vi "Hysteresis-Polynom2Preisach.vi"(9 "Polynomial Coefficients bwd":dbl[](array[numeric]), 10 "relative Range":dbl, 11 "Polynomial Coefficients fwd":dbl[](array[numeric])) -> (3 "Preisach":dbl[](array[numeric]))   [LabVIEW 2016]
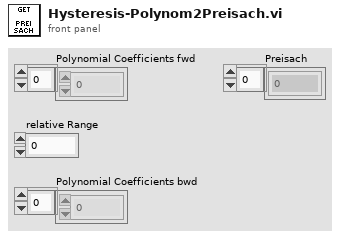
[diagram p1: front panel]
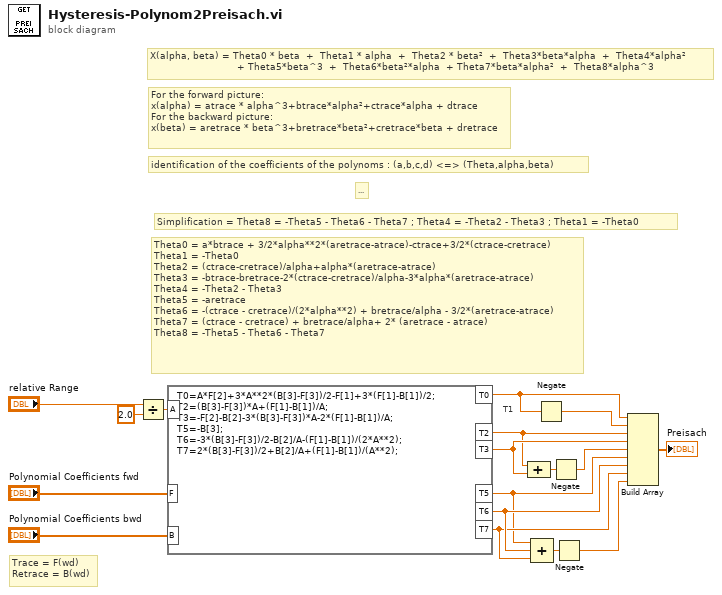
[diagram p0: block diagram]
diagram:
  # "Simplification = Theta8 = -Theta5 - Theta6 - Theta7 ; Theta4 = -Theta2 - Theta3 ; Theta1 = -Theta0"
  # "..."
  # "X(alpha, beta) = Theta0 * beta  +  Theta1 * alpha  +  Theta2 * beta²  +  Theta3*beta*alpha  +  Theta4*alpha² \n                             + Theta5*beta^3  +  Theta6*beta²*alpha  + Theta7*beta*alpha²  +  Theta8*alpha^3"
  # "identification of the coefficients of the polynoms : (a,b,c,d) <=> (Theta,alpha,beta)"
  # "For the forward picture:\nx(alpha) = atrace * alpha^3+btrace*alpha²+ctrace*alpha + dtrace\nFor the backward picture:\nx(beta) = aretrace * beta^3+bretrace*beta²+cretrace*beta + dretrace"
  # "Trace = F(wd)\nRetrace = B(wd)"
  # "T1"
  # "Theta0 = a*btrace + 3/2*alpha**2*(aretrace-atrace)-ctrace+3/2*(ctrace-cretrace)\nTheta1 = -Theta0\nTheta2 = (ctrace-cretrace)/alpha+alpha*(aretrace-atrace)\nTheta3 = -btrace-bretrace-2*(ctrace-cretrace)/alpha-3*alpha*(aretrace-atrace)\nTheta4 = -Theta2 - Theta3\nTheta5 = -aretrace\nTheta6 = -(ctrace - cretrace)/(2*alpha**2) + bretrace/alpha - 3/2*(aretrace-atrace)\nTheta7 = (ctrace - cretrace) + bretrace/alpha+ 2* (aretrace - atrace)\nTheta8 = -Theta5 - Theta6 - Theta7"
  n1 = Divide(x="relative Range", y=2.0) -> (x/y=w17:dbl)
  n2 = formula code="T0=A*F[2]+3*A**2*(B[3]-F[3])/2-F[1]+3*(F[1]-B[1])/2;\nT2=(B[3]-F[3])*A+(F[1]-B[1])/A;\nT3=-F[2]-B[2]-3*(B[3]-F[3])*A-2*(F[1]-B[1])/A;\nT5=-B[3];\nT6=-3*(B[3]-F[3])/2-B[2]/A-(F[1]-B[1])/(2*A**2);\nT7=2*(B[3]-F[3])/2+B[2]/A+(F[1]-B[1])/(A**2);"("A"=w17, "F"="Polynomial Coefficients fwd", "B"="Polynomial Coefficients bwd") -> ("T0"=w7:dbl, "T2"=w2:dbl, "T3"=w3:dbl, "T5"=w10:dbl, "T6"=w12:dbl, "T7"=w11:dbl)
  n3 = Compound Arithmetic op=ADD(w2, w3) -> (w5:dbl)
  n4 = Compound Arithmetic op=ADD(w10, w12, w11) -> (w8:dbl)
  n5 = Negate(x=w7) -> (-x=w6:dbl)
  n6 = Negate(x=w5) -> (-x=w4:dbl)
  n7 = Negate(x=w8) -> (-x=w9:dbl)
  n8 = Build Array(w7, w6, w2, w3, w4, w10, w12, w11, w9) -> (→"Preisach":dbl[])
